vi "Init Encoders.vi"(8 "error in (no error)":errorcluster) -> (0 "error out":errorcluster)   [LabVIEW 2014]
uses:
  <vilib>/Rock Robotics/SystemInterfaces/DIO/FPGA_DIOChannel.ctl
  <vilib>/Rock Robotics/SystemInterfaces/Typedef/FPGA_TypedefDigitalModule.ctl
  <vilib>/Rock Robotics/WPI/Encoder/WPI_EncoderType.ctl
  <vilib>/Rock Robotics/WPI/Counter/WPI_CounterDigitalInputToDigitalSource.vi
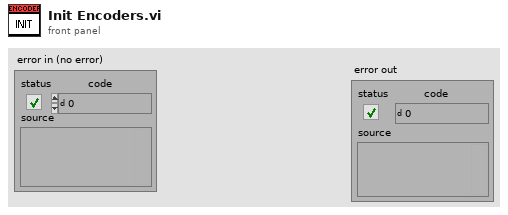
[diagram p1: front panel]
types:
  T1 = typedef "WPI_EncoderType.ctl" = enum16{"1x", "2x", "4x"}
  T2 = typedef "FPGA_TypedefDigitalModule.ctl" = enum16{"Controller 1"}
  T3 = typedef "FPGA_DIOChannel.ctl" = enum8{"DIO 0", "DIO 1", "DIO 2", "DIO 3", "DIO 4", "DIO 5", "DIO 6", "DIO 7", "DIO 8", "DIO 9", "DIO MXP 0", "DIO MXP 1", "DIO MXP 2", "DIO MXP 3", "DIO MXP 4", "DIO MXP 5", "DIO MXP 6", "DIO MXP 7", "DIO MXP 8", "DIO MXP 9", "DIO MXP 10", "DIO MXP 11", "DIO MXP 12", "DIO MXP 13", "DIO MXP 14", "DIO MXP 15", "Invalid"}
  T4 = typedef "WPI_DigitalInputDevRef.ctl" = cluster{"DevStatus":errorcluster, "DIO Channel":T3, "Controller":T2}
  T5 = typedef "FPGA_CounterEncoderSourceConvertionLVSourceType.ctl" = cluster{"DevStatus":errorcluster, "AnalogTriggerMode?":bool, "DigitalMode":cluster{"Controller":T2, "DIO Channel":T6}, "AnalogTriggerMode":cluster{"AnalogTriggerIndex":T7, "OutputType":T8}}
  T6 = typedef "FPGA_DIODigitalSourceChannel.ctl" = enum8{"DIO 0", "DIO 1", "DIO 2", "DIO 3", "DIO 4", "DIO 5", "DIO 6", "DIO 7", "DIO 8", "DIO 9", "DIO MXP 0", "DIO MXP 1", "DIO MXP 2", "DIO MXP 3", "DIO MXP 4", "DIO MXP 5", "DIO MXP 6", "DIO MXP 7", "DIO MXP 8", "DIO MXP 9", "DIO MXP 10", "DIO MXP 11", "DIO MXP 12", "DIO MXP 13", "DIO MXP 14", "DIO MXP 15", "Disabled"}
  T7 = typedef "FPGA_AnalogTriggerIndex.ctl" = enum8{"Trig 0", "Trig 1", "Trig 2", "Trig 3", "Trig 4", "Trig 5", "Trig 6", "Trig 7", "Invalid"}
  T8 = typedef "FPGA_AnalogTriggerOutType.ctl" = enum16{"InWindow", "TriggerState", "Rising", "Falling"}
  T9 = typedef "WPI_EncoderDevRef.ctl" = cluster{"DevStatus":errorcluster, "EncoderIndex":T10, "CounterIndex":T11, "DistancePerCount":dbl, "Decoding Type":T1}
  T10 = typedef "FPGA_EncoderIdx.ctl" = enum8{"Enc 0", "Enc 1", "Enc 2", "Enc 3", "Enc 4", "Enc 5", "Enc 6", "Enc 7", "Invalid"}
  T11 = typedef "FPGA_CounterCtrSystemIndex.ctl" = enum8{"Ctr 0", "Ctr 1", "Ctr 2", "Ctr 3", "Ctr 4", "Ctr 5", "Ctr 6", "Ctr 7", "Invalid"}
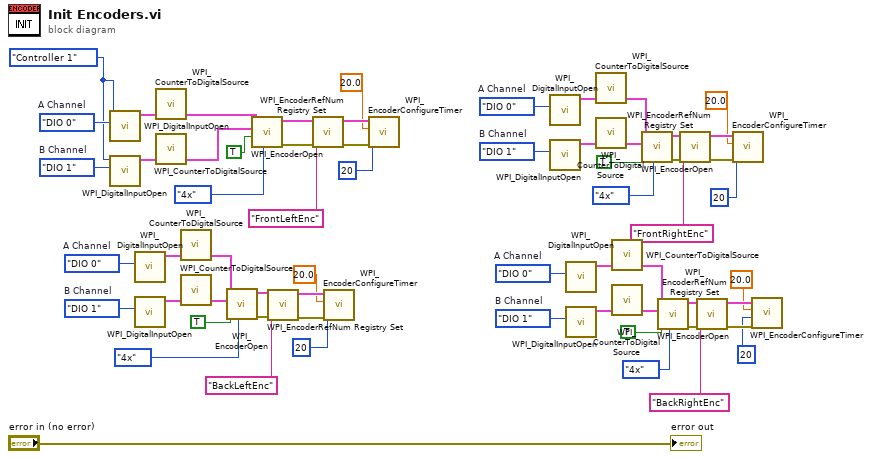
[diagram p0: block diagram]
diagram:
  w13 = FPGA_TypedefDigitalModule."Controller 1" ("Controller")
  w41 = FPGA_DIOChannel."DIO 1"  # B Channel
  w40 = FPGA_DIOChannel."DIO 0"  # A Channel
  w47 = FPGA_DIOChannel."DIO 1"  # B Channel
  w46 = FPGA_DIOChannel."DIO 0"  # A Channel
  w53 = FPGA_DIOChannel."DIO 1"  # B Channel
  w52 = FPGA_DIOChannel."DIO 0"  # A Channel
  w62 = FPGA_DIOChannel."DIO 1"  # B Channel
  w61 = FPGA_DIOChannel."DIO 0"  # A Channel
  n1 = call <vilib>:"WPI_DigitalInputOpen.vi"("DIO Channel"=w61, "Controller"=w13) -> ("DigitalInputDevRef"=w58:T4)  [unwired: 1 in, 8 out]
  n2 = call <vilib>:"WPI_DigitalInputOpen.vi"("DIO Channel"=w62, "Controller"=w13) -> ("DigitalInputDevRef"=w59:T4)  [unwired: 1 in, 8 out]
  n3 = call <vilib>:"WPI_DigitalInputOpen.vi"("DIO Channel"=w52) -> ("DigitalInputDevRef"=w49:T4)  [unwired: 2 in, 8 out]
  n4 = call <vilib>:"WPI_DigitalInputOpen.vi"("DIO Channel"=w53) -> ("DigitalInputDevRef"=w50:T4)  [unwired: 2 in, 8 out]
  n5 = call-poly <vilib>:"WPI_CounterToDigitalSource.vi"("DigitalInputDevRef"=w58) -> ("Digital Source"=w57:T5)  [unwired: 6 out]
  n6 = call-poly <vilib>:"WPI_CounterToDigitalSource.vi"("DigitalInputDevRef"=w59) -> ("Digital Source"=w60:T5)  [unwired: 6 out]
  n7 = call-poly <vilib>:"WPI_CounterToDigitalSource.vi"("DigitalInputDevRef"=w49) -> ("Digital Source"=w48:T5)  [unwired: 6 out]
  n8 = call-poly <vilib>:"WPI_CounterToDigitalSource.vi"("DigitalInputDevRef"=w50) -> ("Digital Source"=w51:T5)  [unwired: 6 out]
  n9 = call <vilib>:"WPI_EncoderOpen.vi"("Decoding Type"=WPI_EncoderType."4x", "Invert Direction (False)"=TRUE, "BSource"=w51, "ASource"=w48) -> ("error out"=w33:errorcluster, "EncoderDevRef"=w32:T9)  [unwired: 4 in, 2 out]
  n10 = call <vilib>:"WPI_EncoderOpen.vi"("Decoding Type"=WPI_EncoderType."4x", "Invert Direction (False)"=TRUE, "BSource"=w60, "ASource"=w57) -> ("error out"=w56:errorcluster, "EncoderDevRef"=w55:T9)  [unwired: 4 in, 2 out]
  n11 = call <vilib>:"WPI_EncoderRefNum Registry Set.vi"("error in (no error)"=w33, "refnum name"="BackLeftEnc", "EncoderDevRef"=w32) -> ("error out"=w21:errorcluster, "EncoderDevRef"=w20:T9)  [unwired: 7 in]
  n12 = call <vilib>:"WPI_EncoderRefNum Registry Set.vi"("error in (no error)"=w56, "refnum name"="FrontLeftEnc", "EncoderDevRef"=w55) -> ("error out"=w17:errorcluster, "EncoderDevRef"=w16:T9)  [unwired: 7 in]
  n13 = call <vilib>:"WPI_EncoderConfigureTimer.vi"("error in (no error)"=w21, "Number Samples to Average"=u8 20, "Minimum Rate"=20.0, "EncoderDevRef"=w20) -> ()  [unwired: 6 in, 2 out]
  n14 = call <vilib>:"WPI_EncoderConfigureTimer.vi"("error in (no error)"=w17, "Number Samples to Average"=u8 20, "Minimum Rate"=20.0, "EncoderDevRef"=w16) -> ()  [unwired: 6 in, 2 out]
  n15 = call <vilib>:"WPI_DigitalInputOpen.vi"("DIO Channel"=w40) -> ("DigitalInputDevRef"=w37:T4)  [unwired: 2 in, 8 out]
  n16 = call <vilib>:"WPI_DigitalInputOpen.vi"("DIO Channel"=w41) -> ("DigitalInputDevRef"=w38:T4)  [unwired: 2 in, 8 out]
  n17 = call <vilib>:"WPI_DigitalInputOpen.vi"("DIO Channel"=w46) -> ("DigitalInputDevRef"=w43:T4)  [unwired: 2 in, 8 out]
  n18 = call <vilib>:"WPI_DigitalInputOpen.vi"("DIO Channel"=w47) -> ("DigitalInputDevRef"=w44:T4)  [unwired: 2 in, 8 out]
  n19 = call-poly <vilib>:"WPI_CounterToDigitalSource.vi"("DigitalInputDevRef"=w37) -> ("Digital Source"=w36:T5)  [unwired: 6 out]
  n20 = call-poly <vilib>:"WPI_CounterToDigitalSource.vi"("DigitalInputDevRef"=w38) -> ("Digital Source"=w39:T5)  [unwired: 6 out]
  n21 = call-poly <vilib>:"WPI_CounterToDigitalSource.vi"("DigitalInputDevRef"=w43) -> ("Digital Source"=w42:T5)  [unwired: 6 out]
  n22 = call-poly <vilib>:"WPI_CounterToDigitalSource.vi"("DigitalInputDevRef"=w44) -> ("Digital Source"=w45:T5)  [unwired: 6 out]
  n23 = call <vilib>:"WPI_EncoderOpen.vi"("Decoding Type"=WPI_EncoderType."4x", "Invert Direction (False)"=TRUE, "BSource"=w39, "ASource"=w36) -> ("error out"=w35:errorcluster, "EncoderDevRef"=w34:T9)  [unwired: 4 in, 2 out]
  n24 = call <vilib>:"WPI_EncoderOpen.vi"("Decoding Type"=WPI_EncoderType."4x", "Invert Direction (False)"=TRUE, "BSource"=w45, "ASource"=w42) -> ("error out"=w31:errorcluster, "EncoderDevRef"=w30:T9)  [unwired: 4 in, 2 out]
  n25 = call <vilib>:"WPI_EncoderRefNum Registry Set.vi"("error in (no error)"=w35, "refnum name"="FrontRightEnc", "EncoderDevRef"=w34) -> ("error out"=w12:errorcluster, "EncoderDevRef"=w11:T9)  [unwired: 7 in]
  n26 = call <vilib>:"WPI_EncoderRefNum Registry Set.vi"("error in (no error)"=w31, "refnum name"="BackRightEnc", "EncoderDevRef"=w30) -> ("error out"=w5:errorcluster, "EncoderDevRef"=w6:T9)  [unwired: 7 in]
  n27 = call <vilib>:"WPI_EncoderConfigureTimer.vi"("error in (no error)"=w12, "Number Samples to Average"=u8 20, "Minimum Rate"=20.0, "EncoderDevRef"=w11) -> ()  [unwired: 6 in, 2 out]
  n28 = call <vilib>:"WPI_EncoderConfigureTimer.vi"("error in (no error)"=w5, "Number Samples to Average"=u8 20, "Minimum Rate"=20.0, "EncoderDevRef"=w6) -> ()  [unwired: 6 in, 2 out]
  "error out" <- "error in (no error)"
